vi "Image Get Line ROI Extremities.vi"(8 "Error In":errorcluster, 11 "ROI":T2) -> (0 "Error Out":errorcluster, 1 "Is Line?":bool, 3 "Line Extremities":T1[](array[typedef]))   [LabVIEW 2021, in "Image.lvlib"]
uses:
  Image.lvlib
  Image Point.ctl
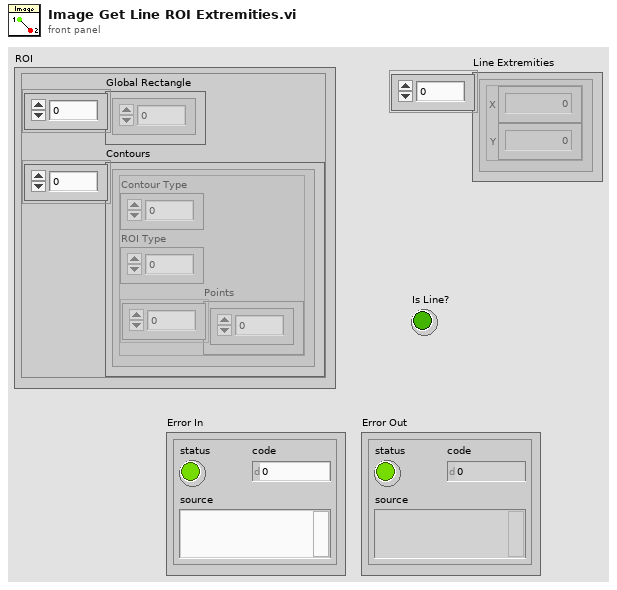
[diagram p1: front panel]
types:
  T1 = typedef "Image.lvlib/Image Point.ctl" = cluster{"X":i32, "Y":i32}
  T2 = cluster{"Global Rectangle":i32[], "Contours":cluster{"Contour Type":u32, "ROI Type":u32, "Points":i32[]}[]}
  T3 = cluster{"Contour Type":u32, "ROI Type":u32, "Points":i32[]}[]
  T4 = cluster{"Contour Type":u32, "ROI Type":u32, "Points":i32[]}
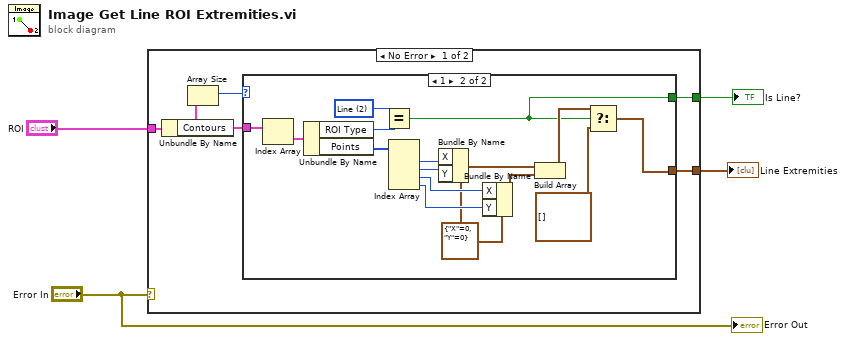
[diagram p0: block diagram]
diagram:
  n1 = case shown="No Error" "Error In" {
    tunnel: "ROI" -> [w9 _]
    tunnel: [w6 _] -> w3
    tunnel: [w5 _] -> w1
    frame No Error {
      n2 = Unbundle By Name(w9) -> ("Contours"=w7:T3)
      n3 = Array Size(array=w7) -> (size(s)=w8:i32)
      n4 = case shown="1" w8 {
        tunnel: w7 -> [_ w25]
        tunnel: [_ w12] -> w6
        tunnel: [_ w10] -> w5
        frame 0, Default {
        }
        frame 1 {
          w16 = T1 {"X"=0, "Y"=0} ("Image Point")
          w23 = u32 2 items=["No Selection", "Point", "Line", "Rectangle", "Oval", "Polygon", "Freehand Region", "Annulus", "Unused2", "Unused3", "Broken Line", "Freehand Line", "Rotated Rectangle"] ("Type")
          n5 = Index Array(array=w25) -> (element=w24:T4)  [unwired: 1 in]
          n6 = Unbundle By Name(w24) -> ("ROI Type"=w22:u32, "Points"=w21:i32[])
          n7 = Equal?(x=w23, y=w22) -> (x = y?=w10:bool)
          n8 = Index Array(array=w21) -> (element #1=w20:i32, element #2=w19:i32, element #3=w18:i32, element #4=w17:i32)  [unwired: 4 in]
          n9 = Bundle By Name(cluster=w16, "X"=w20, "Y"=w19) -> (w15:T1)
          n10 = Bundle By Name(cluster=w16, "X"=w18, "Y"=w17) -> (w14:T1)
          n11 = Build Array(w15, w14) -> (w13:T1[])
          n12 = Select(t=w13, s=w10, f=T1[] []) -> (s? t:f=w12:T1[])
        }
      }
    }
    frame Error {
    }
  }
  "Line Extremities" <- w3
  "Is Line?" <- w1
  "Error Out" <- "Error In"
